vi "Preset STEP HOLD time.vi"(8 "error in (no error)":errorcluster, 10 "Time":dbl=0.2 min=0.1 max=99.9 step=0.1 format="%.1g", 11 "VISA resource in":refnum<visa-resource-name>) -> (0 "error out":errorcluster, 3 "VISA resource out":refnum<visa-resource-name>)   [LabVIEW 2025, in "Chroma 19572.lvlib"]
doc: "This VI writes to the instrument the STEP HOLD time."
uses:
  <instrlib>/Chroma 19572/Chroma 19572.lvlib
panel:
  # "[sec]"
  # "PreSet STEP HOLD time"
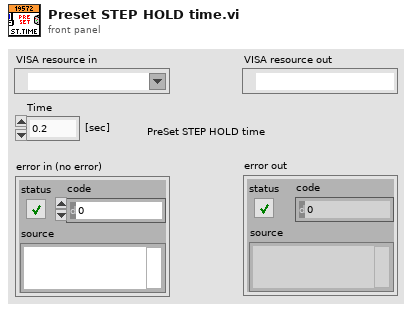
[diagram p1: front panel]
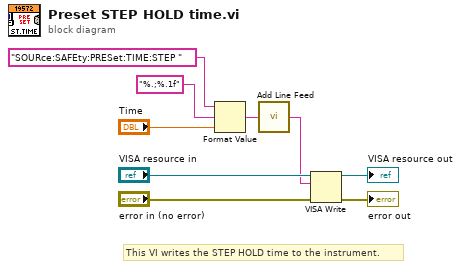
[diagram p0: block diagram]
diagram:
  # "This VI writes the STEP HOLD time to the instrument."
  n1 = Format Value(string ("")="SOURce:SAFEty:PRESet:TIME:STEP ", format string="%.;%.1f", value (0)="Time") -> (output string=w3:string)
  n2 = call <instrlib>:"Add Line Feed.vi"("Command string"=w3) -> ("Concatenated string"=w5:string)  [unwired: 4 in]
  n3 = VISA Write(VISA resource name="VISA resource in", write buffer=w5, error in (no error)="error in (no error)") -> (VISA resource name out=→"VISA resource out":refnum<visa-resource-name>, error out=→"error out":errorcluster)  [unwired: 1 out]
